vi "Smart_Garden.vi"() -> ()   [LabVIEW 2020]
panel:
  out "?":bool
  out "?":bool
  out "?":bool
  out "?":bool
  out "?":bool
  out "?":bool
  out "?":bool
  out "?":bool
  out "?":bool
  out "?":bool
  out "?":bool
  out "?":bool
  out "?":bool
  out "?":bool
  out "?":bool
  out "?":bool
  out "?":bool
  out "?":bool
  out "?":bool
  out "?":bool
  out "?":bool
  out "?":bool
  out "?":bool
  out "?":bool
  out "?":bool
  out "?":bool
  in  "?":bool
  out "Max":string
  out "Min":string
  out "Max":string
  out "Min":string
  out "Max":string
  out "Min":string
  out "Min":string
  out "Max":string
  in  "Water":dbl(slide) scale=0.0..100.0
  in  "?":i32
  out "Water lvl \nsensor":dbl(slide) scale=0.0..100.0
  in  "Run":bool
  in  "Capacity":dbl min=0.0 max=100.0 format="%#_3g"
  out "Window":bool
  out "Co2  Supply":bool
  out "Co2 condition":string
  out "Co2 \nWARNING!!":bool
  out "Co2 sensor":dbl(knob) scale=0.0..1300.0
  in  "Co2 (ppm)":dbl(knob) scale=0.0..1300.0
  in  "Range":i32=5
  out "Timer":i32
  out "Grow Light":bool
  out "Sun shade":bool
  in  "Run":bool
  out "Lux condition":string
  out "Lux WARNING!!":bool
  out "Lux sensor":sgl(knob) scale=0.0..30000.0
  in  "Light (lux)":dbl(slide) scale=0.0..30000.0
  out "Space\nHeater":bool
  out "Fan":bool
  out "Temp condition":string
  in  "Temp (C)":dbl(slide) scale=0.0..40.0
  out "Temp \nWARNING!!":bool
  out "Temp sensor":sgl(slide) scale=0.0..40.0
  out "pH condition":string
  in  "pH lvl":dbl(slide) scale=0.0..10.0 scale format="%#_2g"
  out "pH WARNING!!":bool
  out "pH sensor":sgl(slide) scale=0.0..10.0
  # "PEJAL"
  # "AZRUL"
  # "DERRICK"
  # "MIMI"
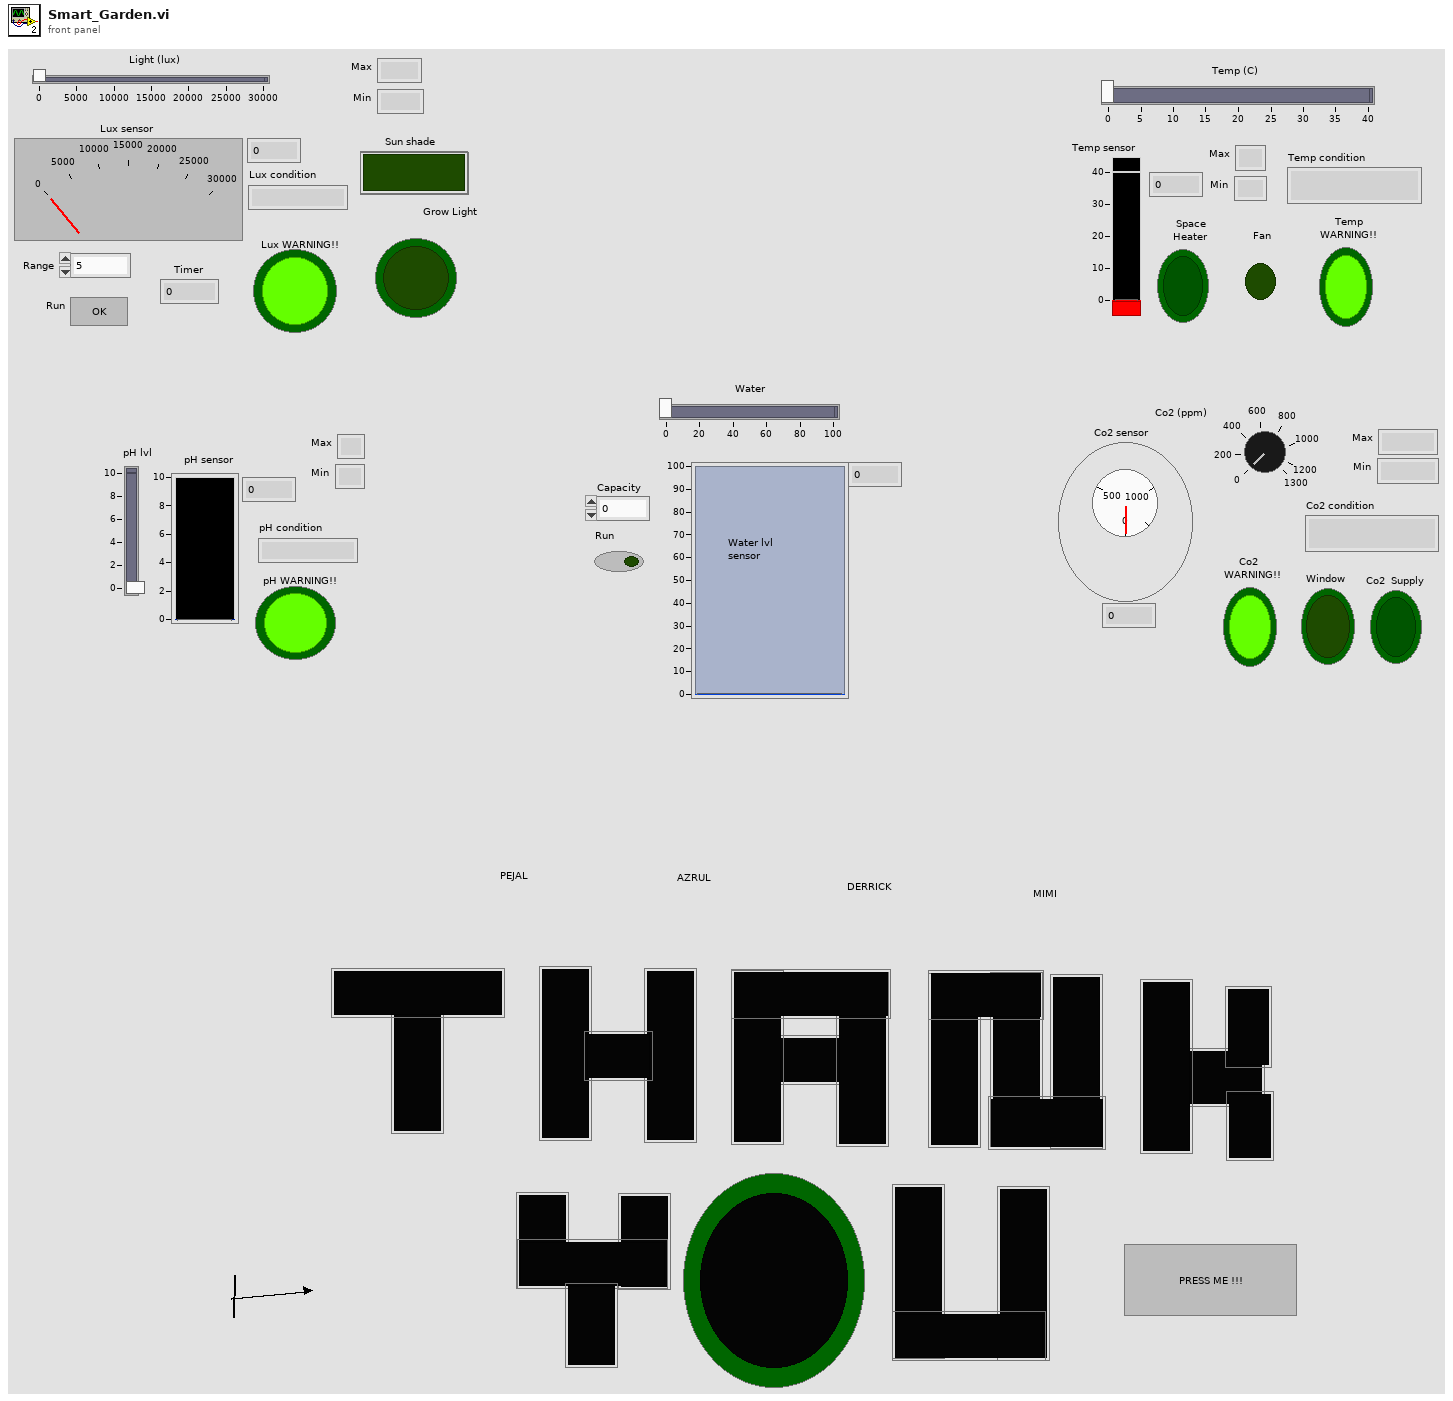
[diagram p1: front panel]
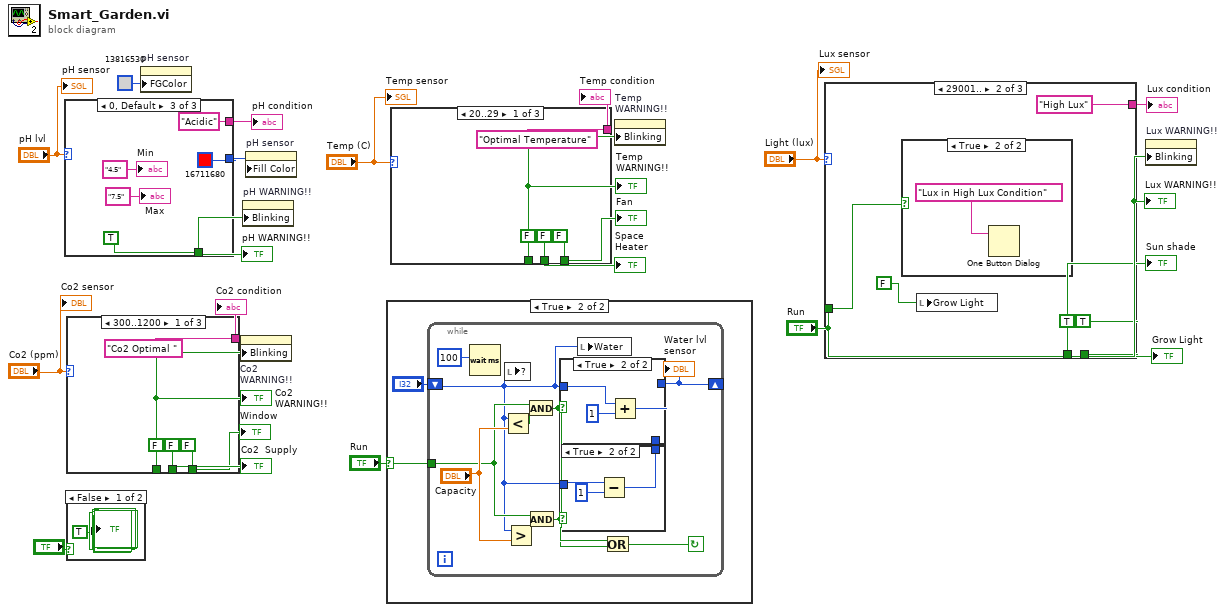
[diagram p0: block diagram]
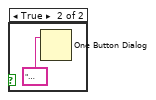
[diagram p2: hidden frame]
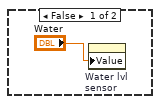
[diagram p3: hidden frame]
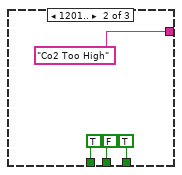
[diagram p6: hidden frame]
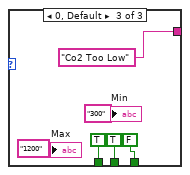
[diagram p7: hidden frame]
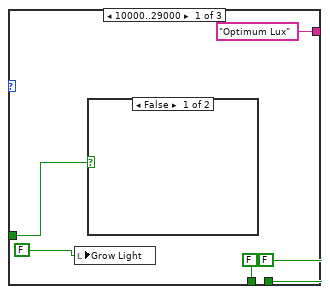
[diagram p8: hidden frame]
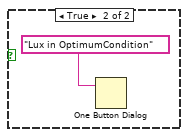
[diagram p9: hidden frame]
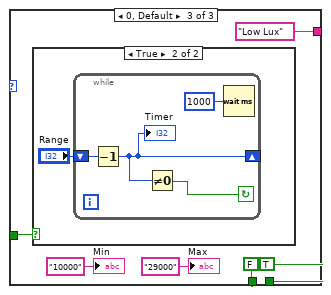
[diagram p11: hidden frame]
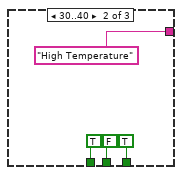
[diagram p13: hidden frame]
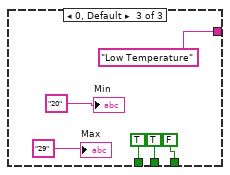
[diagram p14: hidden frame]
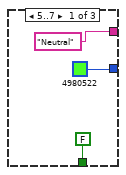
[diagram p15: hidden frame]
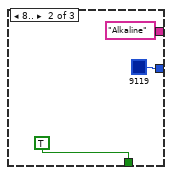
[diagram p16: hidden frame]
diagram:
  n1 = case shown="0, Default" "pH lvl" {
    tunnel: [u32 4980522 ("Fill Color") u32 9119 ("Fill Color") u32 16711680 ("Housing Colors:FG Color")] -> w14
    tunnel: [FALSE TRUE TRUE] -> w15
    tunnel: ["Neutral" "Alkaline" "Acidic"] -> w16
    frame 5..7 {
    }
    frame 8.. {
    }
    frame 0, Default {
      "Min" <- "4.5" ("Max")
      "Max" <- "7.5" ("Max")
    }
  }
  "pH WARNING!!" <- w15
  "pH condition" <- w16
  n2 = case shown="300..1200" "Co2 (ppm)" {
    tunnel: [FALSE TRUE TRUE] -> w6
    tunnel: ["Co2 Optimal " "Co2 Too High" "Co2 Too Low"] -> w8
    tunnel: [FALSE TRUE FALSE] -> w4
    tunnel: [FALSE FALSE TRUE] -> w7
    frame 300..1200 {
    }
    frame 1201.. {
    }
    frame 0, Default {
      "Min" <- "300" ("Max")
      "Max" <- "1200" ("Max")
    }
  }
  "Co2 \nWARNING!!" <- w6
  "Co2 condition" <- w8
  "Co2  Supply" <- w7
  "Window" <- w4
  n3 = case shown="False" "?" {
    frame False {
      w48 = TRUE
      "?" <- w48
      "?" <- w48
      "?" <- w48
      "?" <- w48
      "?" <- w48
      "?" <- w48
      "?" <- w48
      "?" <- w48
      "?" <- w48
      "?" <- w48
      "?" <- w48
      "?" <- w48
      "?" <- w48
      "?" <- w48
      "?" <- w48
      "?" <- w48
      "?" <- w48
      "?" <- w48
      "?" <- w48
      "?" <- w48
      "?" <- w48
      "?" <- w48
      "?" <- w48
      "?" <- w48
      "?" <- w48
      "?" <- w48
    }
    frame True {
      n4 = One Button Dialog(message="                       SMART GARDEN PROJECT\n\nPREPARED BY:\n\nMUHAMMAD AZRUL BIN REDZUAN      (B122310626)  \n \nDANISH HAMIMI BIN NORHISHAM       (B122310625)  \n \nFAISAL HAQIEM BIN FIRDAUS                 (B122310 031)         \n                        \nDERRICK CHONG JUN CHI                        (B122310578)\n\n\n\nPREPARED FOR: \n\n              SIR FAREES EZWAN BIN MOHD SANI\n\n   ") -> ()  [unwired: 1 in, 1 out]
    }
  }
  n5 = property on="pH sensor" class="Slide (strict)"("FGColor"=u32 13816530 ("Housing Colors:FG Color")) -> ()  [unwired: 2 in, 2 out]
  n6 = property on="Co2 \nWARNING!!" class="Bool (strict)"("Blinking"=w6) -> ()  [unwired: 2 in, 2 out]
  n7 = property on="pH WARNING!!" class="Bool (strict)"("Blinking"=w15) -> ()  [unwired: 2 in, 2 out]
  n8 = property on="pH sensor" class="Slide (strict)"("Fill Color"=w14) -> ()  [unwired: 2 in, 2 out]
  n9 = case shown="True" "Run" {
    selector: "Run" -> [_ w51]
    frame False {
      n10 = property on="Water lvl \nsensor" class="Slide (strict)"("Value"="Water") -> ()  [unwired: 2 in, 2 out]
    }
    frame True {
      n11 = while {
        shift-right: [w59] -> _
        shift-left: "?" -> [w53]
        tunnel: w51 -> [w58]
        stop <- w57 continue-if-true
        n12 = Wait (ms)(milliseconds to wait=u32 100) -> ()  [unwired: 1 out]
        n13 = Less?(x=w53, y="Capacity") -> (x < y?=w63:bool)
        n14 = local write item#28(w53) -> ()
        n15 = Greater?(x=w53, y="Capacity") -> (0:w62:bool)
        n16 = And(x=w58, y=w63) -> (x .and. y?=w56:bool)
        n17 = And(x=w58, y=w62) -> (x .and. y?=w55:bool)
        n18 = case shown="True" w55 {
          tunnel: w53 -> [w64 w67]
          tunnel: [w64 w65] -> w61
          frame False {
          }
          frame True {
            n19 = Subtract(x=w67, y=1) -> (x-y=w65:i32)
          }
        }
        n20 = case shown="True" w56 {
          tunnel: w53 -> [_ w71]
          tunnel: [w68 w69] -> w59
          tunnel: w61 -> [w68 _]
          frame False {
          }
          frame True {
            n21 = Add(x=w71, y=1) -> (x+y=w69:i32)
          }
        }
        "Water lvl \nsensor" <- w59
        n22 = local write "Water"(w53) -> ()
        n23 = Or(x=w56, y=w55) -> (x .or. y?=w57:bool)
      }
    }
  }
  n24 = case shown="20..29" "Temp (C)" {
    tunnel: [FALSE TRUE TRUE] -> w18
    tunnel: ["Optimal Temperature" "High Temperature" "Low Temperature"] -> w22
    tunnel: [FALSE TRUE FALSE] -> w20
    tunnel: [FALSE FALSE TRUE] -> w21
    frame 20..29 {
    }
    frame 30..40 {
    }
    frame 0, Default {
      "Min" <- "20" ("Max")
      "Max" <- "29" ("Max")
    }
  }
  "Temp \nWARNING!!" <- w18
  "Temp condition" <- w22
  "Fan" <- w20
  "Space\nHeater" <- w21
  n25 = property on="Temp \nWARNING!!" class="Bool (strict)"("Blinking"=w18) -> ()  [unwired: 2 in, 2 out]
  n26 = case shown="29001.." "Light (lux)" {
    tunnel: ["Optimum Lux" "High Lux" "Low Lux"] -> w12
    tunnel: [FALSE TRUE TRUE] -> w10
    tunnel: [FALSE TRUE FALSE] -> w9
    tunnel: "Run" -> [w87 w92 w100]
    frame 10000..29000 {
      n27 = local write "Grow Light"(FALSE) -> ()
      n28 = case shown="False" w87 {
        frame False {
        }
        frame True {
          n29 = One Button Dialog(message="Lux in OptimumCondition") -> ()  [unwired: 1 in, 1 out]
        }
      }
    }
    frame 29001.. {
      n30 = case shown="True" w92 {
        frame False {
        }
        frame True {
          n31 = One Button Dialog(message="Lux in High Lux Condition") -> ()  [unwired: 1 in, 1 out]
        }
      }
      n32 = local write "Grow Light"(FALSE) -> ()
    }
    frame 0, Default {
      n33 = case shown="True" w100 {
        frame False {
        }
        frame True {
          n34 = while {
            shift-right: [w106] -> _
            shift-left: "Range" -> [w107]
            stop <- w105 continue-if-true
            n35 = Decrement(x=w107) -> (x-1=w106:i32)
            "Timer" <- w106
            n36 = Not Equal To 0?(x=w106) -> (x != 0?=w105:bool)
            n37 = Wait (ms)(milliseconds to wait=u32 1000) -> ()  [unwired: 1 out]
          }
        }
      }
      "Min" <- "10000" ("Max")
      "Max" <- "29000" ("Max")
    }
  }
  "Lux WARNING!!" <- w10
  "Lux condition" <- w12
  "Sun shade" <- w9
  n38 = property on="Lux WARNING!!" class="Bool (strict)"("Blinking"=w10) -> ()  [unwired: 2 in, 2 out]
  "pH sensor" <- "pH lvl"
  "Temp sensor" <- "Temp (C)"
  "Lux sensor" <- "Light (lux)"
  "Grow Light" <- "Run"
  "Co2 sensor" <- "Co2 (ppm)"
